vi "Shutdown Module.vi"(8 "error in (no error)":errorcluster, 9 "params":variant, 11 "Controller in":refnum<class "Controller.lvclass">) -> (0 "error out":errorcluster, 3 "Controller out":refnum<class "Controller.lvclass">)   [LabVIEW 2020, in "Controller.lvclass"]
uses:
  Controller.lvclass
  Controller.lvclass/Controller.ctl
  Module/Module.lvclass
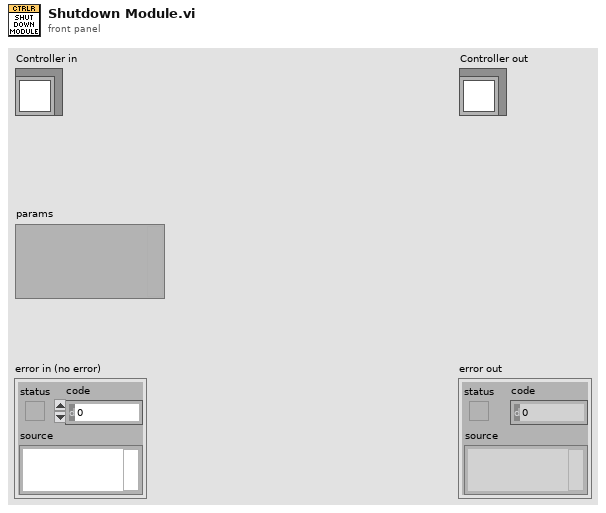
[diagram p1: front panel]
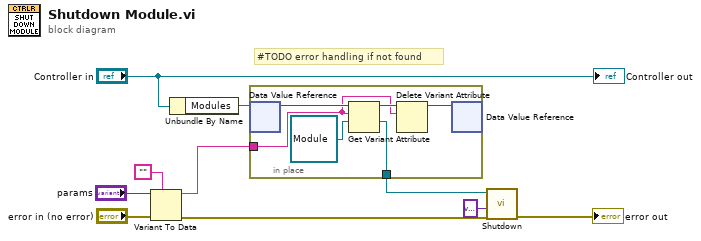
[diagram p0: block diagram]
diagram:
  # "#TODO error handling if not found"
  n1 = Variant To Data(error in="error in (no error)", type="", Variant="params") -> (data=w2:string, error out=w4:errorcluster)
  n2 = Unbundle By Name("Controller in") -> ("Modules"=w8:refnum<data-value>)
  n3 = in-place {
    in-place-border: w2 -> [w11]
    in-place-border: [w12] -> w7
    n4 = in-place-dvr #1(w8) -> (w15:variant)  [unwired: 1 out]
    n5 = Get Variant Attribute(Variant=w15, name=w11, default value (empty Variant)=refnum<class "Module.lvclass"> refnum ("Module.lvclass")) -> (duplicate Variant=w14:variant, value=w12:refnum<class "Module.lvclass">)  [unwired: 1 in, 2 out]
    n6 = Delete Variant Attribute(6:w11, 7:w14) -> (3:w16:variant)  [unwired: 1 in, 2 out]
    n7 = in-place-dvr #1(w16) -> ()  [unwired: 2 out]
  }
  n8 = call "Shutdown.vi"("error in (no error)"=w4, "Params"=variant ("Message Data"), "Module in"=w7) -> ("error out"=→"error out":errorcluster)  [unwired: 7 in, 1 out]
  "Controller out" <- "Controller in"
